vi "02guarda_paneles_file.vi"(0 "Paneles":T2(array[cluster]) {"Numeric" min=1.0 max=60.0 step=1.0 format="%#2.1f"; "Ultima recepción" format="%<%d/%m - %X>T"; "Med\nPpal" format="%_4g"}, 1 "Block":bool=TRUE, 2 "data path":string, 3 "Cant equipos":u8(ring)=30 items=["30"=30, "36"=36, "42"=42, "48"=48, "54"=54, "60"=60], 4 "Sound?":bool caption="SONIDO", 6 "Config Equipos":T1(array[cluster])=[{"Modelo"="", "IP"="", "Puerto"=0, "Time Out"=0, "Med Princ"=0, "Time sin rx"=60, "Reintento"=60, "Ref PD"=200}] {"Ref PD" max=10000 step=1; "Med Princ" items=["1", "2", "3", "4", "5", "6", "7", "8", "9", "10", "11", "12", "13", "14", "15", "16", "17", "18", "19", "20", "21", "22", "23", "24", "25", "26", "27", "28", "29", "30", "31", "32"]}) -> (5 "error out":errorcluster)   [LabVIEW 2010]
uses:
  <vilib>/Utility/file.llb/Write To Spreadsheet File (I64).vi
  <vilib>/Utility/file.llb/Write To Spreadsheet File (string).vi
  <vilib>/Utility/file.llb/Write To Spreadsheet File (DBL).vi
panel:
  out "Alarmas":i64[](array[numeric])
  out "Nombre paneles":string[](array[string])
  out "Time paneles":dbl[](array[numeric])
  out "Estado paneles":i64[](array[numeric])
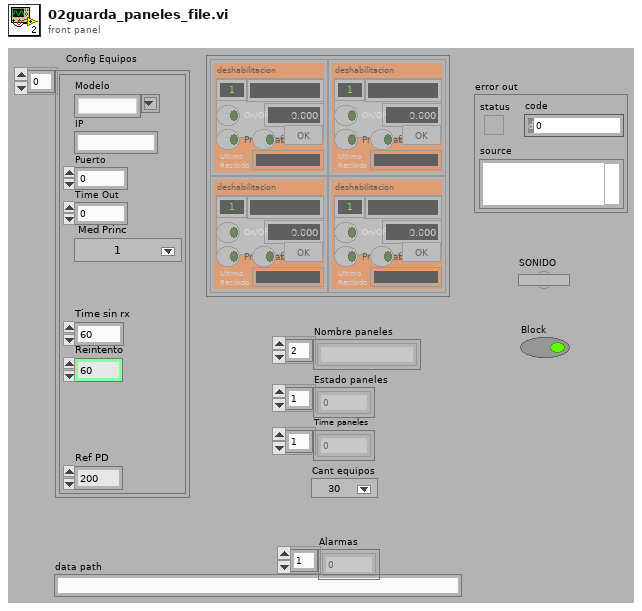
[diagram p1: front panel]
types:
  T1 = cluster{"Modelo":string, "IP":string, "Puerto":u16, "Time Out":u16, "Med Princ":u16, "Time sin rx":u16, "Reintento":u16, "Ref PD":u16}[]
  T2 = cluster{"Nombre":string, "Med\nPpal":dbl, "On/Off":bool, "Ultima recepción":timestamp, "Numeric":dbl, "deshabilitacion":bool, "Prioridad":bool, "falla":bool, "alarm":bool}[][]
  T3 = enum16{"open", "replace", "create", "open or create", "replace or create", "replace or create with confirmation"}
  T4 = cluster{"Nombre":string, "Med\nPpal":dbl, "On/Off":bool, "Ultima recepción":timestamp, "Numeric":dbl, "deshabilitacion":bool, "Prioridad":bool, "falla":bool, "alarm":bool}
  T5 = cluster{"Modelo":string, "IP":string, "Puerto":u16, "Time Out":u16, "Med Princ":u16, "Time sin rx":u16, "Reintento":u16, "Ref PD":u16}
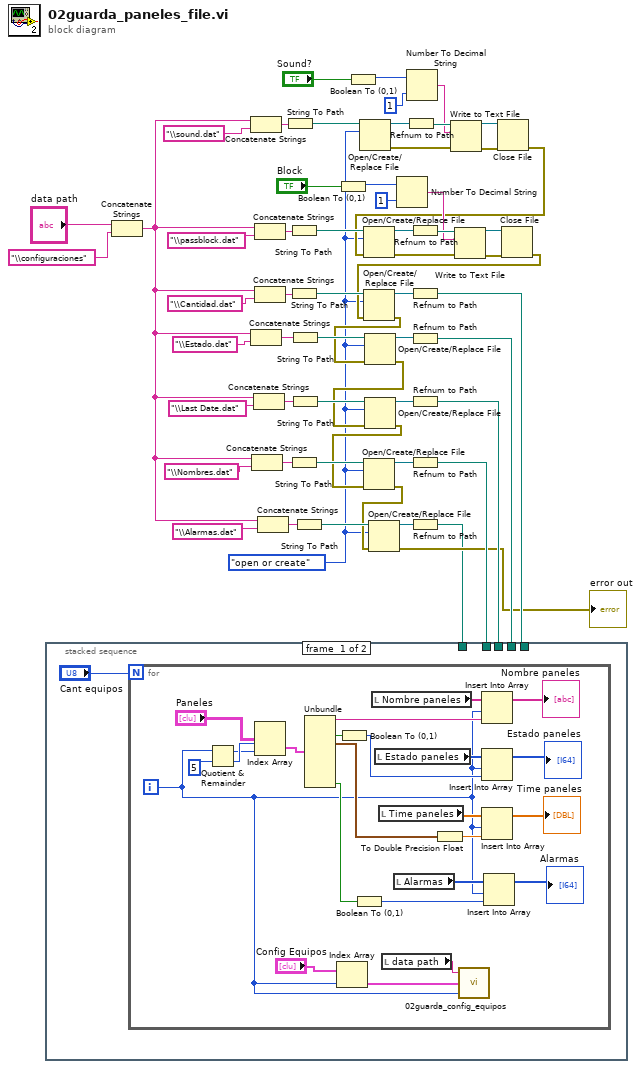
[diagram p0: block diagram]
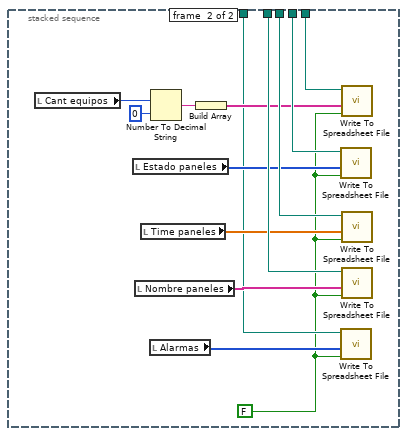
[diagram p2: hidden frame]
diagram:
  w3 = T3."open or create" ("operation (0:open)")
  n1 = Concatenate Strings("data path", "\\configuraciones") -> (w2:string)
  n2 = Concatenate Strings(w2, "\\sound.dat") -> (w7:string)
  n3 = Concatenate Strings(w2, "\\Estado.dat") -> (w56:string)
  n4 = Concatenate Strings(w2, "\\Nombres.dat") -> (w57:string)
  n5 = Concatenate Strings(w2, "\\Last Date.dat") -> (w55:string)
  n6 = Concatenate Strings(w2, "\\passblock.dat") -> (w35:string)
  n7 = Concatenate Strings(w2, "\\Cantidad.dat") -> (w44:string)
  n8 = Concatenate Strings(w2, "\\Alarmas.dat") -> (w21:string)
  n9 = String To Path(string=w7) -> (path=w8:path)
  n10 = String To Path(string=w35) -> (path=w34:path)
  n11 = String To Path(string=w44) -> (path=w45:path)
  n12 = String To Path(string=w57) -> (path=w52:path)
  n13 = String To Path(string=w56) -> (path=w53:path)
  n14 = String To Path(string=w55) -> (path=w54:path)
  n15 = String To Path(string=w21) -> (path=w20:path)
  n16 = Boolean To (0,1)(Boolean="Block") -> (0, 1=w27:i16)
  n17 = Boolean To (0,1)(Boolean="Sound?") -> (0, 1=w14:i16)
  n18 = Open/Create/Replace File(file path (use dialog)=w8, operation (0:open)=w3) -> (refnum out=w5:refnum<file>, error out=w11:errorcluster)  [unwired: 1 in, 4 out]
  n19 = Number To Decimal String(number=w27, width (-)=i16 1) -> (decimal integer string=w25:string)
  n20 = Refnum to Path(1:w5) -> (0:w9:path)
  n21 = Number To Decimal String(number=w14, width (-)=i16 1) -> (decimal integer string=w1:string)
  n22 = Write to Text File(file (use dialog)=w9, text=w1, error in=w11) -> (refnum out=w10:refnum<file>, error out=w12:errorcluster)  [unwired: 1 in, 1 out]
  n23 = Close File(refnum=w10, error in=w12) -> (error out=w4:errorcluster)  [unwired: 1 out]
  n24 = Open/Create/Replace File(file path (use dialog)=w34, error in=w4, operation (0:open)=w3) -> (refnum out=w37:refnum<file>, error out=w31:errorcluster)  [unwired: 4 out]
  n25 = Refnum to Path(1:w37) -> (0:w33:path)
  n26 = Write to Text File(file (use dialog)=w33, text=w25, error in=w31) -> (refnum out=w32:refnum<file>, error out=w30:errorcluster)  [unwired: 1 in, 1 out]
  n27 = Close File(refnum=w32, error in=w30) -> (error out=w29:errorcluster)  [unwired: 1 out]
  n28 = Open/Create/Replace File(file path (use dialog)=w45, error in=w29, operation (0:open)=w3) -> (refnum out=w42:refnum<file>, error out=w39:errorcluster)  [unwired: 4 out]
  n29 = Open/Create/Replace File(file path (use dialog)=w53, error in=w39, operation (0:open)=w3) -> (refnum out=w49:refnum<file>, error out=w40:errorcluster)  [unwired: 4 out]
  n30 = Open/Create/Replace File(file path (use dialog)=w54, error in=w40, operation (0:open)=w3) -> (refnum out=w48:refnum<file>, error out=w38:errorcluster)  [unwired: 4 out]
  n31 = Open/Create/Replace File(file path (use dialog)=w52, error in=w38, operation (0:open)=w3) -> (refnum out=w51:refnum<file>, error out=w16:errorcluster)  [unwired: 4 out]
  n32 = Open/Create/Replace File(file path (use dialog)=w20, error in=w16, operation (0:open)=w3) -> (refnum out=w19:refnum<file>, error out=→"error out":errorcluster)  [unwired: 4 out]
  n33 = Refnum to Path(1:w42) -> (0:w41:path)
  n34 = Refnum to Path(1:w49) -> (0:w47:path)
  n35 = Refnum to Path(1:w48) -> (0:w46:path)
  n36 = Refnum to Path(1:w51) -> (0:w50:path)
  n37 = Refnum to Path(1:w19) -> (0:w17:path)
  n38 = stacked-sequence {
    tunnel: w50 -> [_ w99]
    tunnel: w47 -> [_ w97]
    tunnel: w46 -> [_ w96]
    tunnel: w41 -> [_ w91]
    tunnel: w17 -> [_ w87]
    frame #0 {
      n39 = for {
        N: "Cant equipos" -> [_]
        i -> [w62]
        n40 = Quotient & Remainder(x=w62, y=5) -> (x-y*floor(x/y)=w70:i32, floor(x/y)=w71:i32)
        n41 = Index Array(array="Paneles", index (row)=w71, index (col)=w70) -> (element=w68:T4)
        n42 = Unbundle(w68) -> ("Nombre"=w85:string, "On/Off"=w77:bool, "Ultima recepción"=w81:timestamp, "alarm"=w63:bool)  [unwired: 5 out]
        n43 = Index Array(array="Config Equipos", index=w62) -> (element=w73:T5)
        n44 = Boolean To (0,1)(Boolean=w77) -> (0, 1=w76:i16)
        n45 = Boolean To (0,1)(Boolean=w63) -> (0, 1=w65:i16)
        n46 = local read "Nombre paneles"() -> (w83:string[])
        n47 = local read "Estado paneles"() -> (w78:i64[])
        n48 = local read "Time paneles"() -> (w79:dbl[])
        n49 = local read "data path"() -> (w74:string)
        n50 = local read "Alarmas"() -> (w66:i64[])
        n51 = To Double Precision Float(number=w81) -> (double precision float=w82:dbl)
        n52 = call "02guarda_config_equipos.vi"("Nº equipo"=w62, "Config equipo"=w73, "exe path"=w74) -> ()  [unwired: 1 out]
        n53 = Insert Into Array(array=w83, index=w62, new element=w85) -> (→"Nombre paneles":string[])
        n54 = Insert Into Array(array=w78, index=w62, new element=w76) -> (→"Estado paneles":i64[])
        n55 = Insert Into Array(array=w79, index=w62, new element=w82) -> (→"Time paneles":dbl[])
        n56 = Insert Into Array(array=w66, index=w62, new element=w65) -> (→"Alarmas":i64[])
      }
    }
    frame #1 {
      w86 = FALSE ("append to file? (new file:F)")
      n57 = local read "Cant equipos"() -> (w93:u8)
      n58 = local read "Estado paneles"() -> (w94:i64[])
      n59 = local read "Nombre paneles"() -> (w98:string[])
      n60 = local read "Time paneles"() -> (w95:dbl[])
      n61 = local read "Alarmas"() -> (w88:i64[])
      n62 = Number To Decimal String(number=w93, width (-)=i16 0) -> (decimal integer string=w90:string)
      n63 = Build Array(w90) -> (w89:string[])
      n64 = call-poly <vilib>:"Write To Spreadsheet File.vi"("append to file? (new file:F)"=w86, "1D data"=w94, "file path (dialog if empty)"=w97) -> ()  [unwired: 3 in, 3 out]
      n65 = call-poly <vilib>:"Write To Spreadsheet File.vi"("append to file? (new file:F)"=w86, "1D data"=w88, "file path (dialog if empty)"=w87) -> ()  [unwired: 3 in, 3 out]
      n66 = call-poly <vilib>:"Write To Spreadsheet File.vi"("append to file? (new file:F)"=w86, "1D data"=w89, "file path (dialog if empty)"=w91) -> ()  [unwired: 3 in, 3 out]
      n67 = call-poly <vilib>:"Write To Spreadsheet File.vi"("append to file? (new file:F)"=w86, "1D data"=w95, "file path (dialog if empty)"=w96) -> ()  [unwired: 3 in, 3 out]
      n68 = call-poly <vilib>:"Write To Spreadsheet File.vi"("append to file? (new file:F)"=w86, "1D data"=w98, "file path (dialog if empty)"=w99) -> ()  [unwired: 3 in, 3 out]
    }
  }
